vi "Close.vi"(8 "error in (no error)":errorcluster, 11 "VideoMux in":refnum<class "VideoMux.lvclass">) -> (0 "error out":errorcluster)   [LabVIEW 2022 SP3, in "VideoMux.lvlib" / "VideoMux.lvclass"]
uses:
  VideoMux.lvclass
  VideoMux.lvclass/VideoMux.ctl
  <vilib>/IlluminatedG/IG HTTP Server/HTTP Server/Server/Server.lvclass
  <vilib>/ActorFramework/Stop Msg/Stop Msg.lvclass
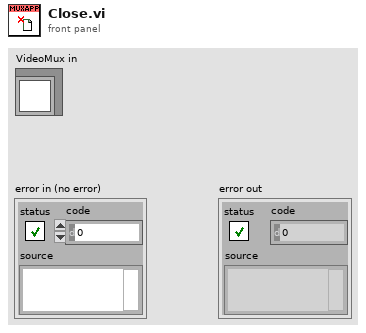
[diagram p1: front panel]
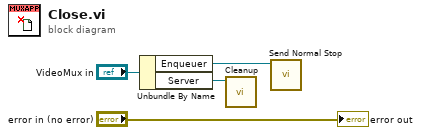
[diagram p0: block diagram]
diagram:
  n1 = Unbundle By Name("VideoMux in") -> ("Enqueuer"=w1:refnum<class "Message Enqueuer.lvclass">, "Server"=w2:refnum<class "Server.lvclass">)
  n2 = call <vilib>:"Cleanup.vi"("Server in"=w2) -> ()  [unwired: 10 in, 1 out]
  n3 = call <vilib>:"Send Normal Stop.vi"("Message Enqueuer"=w1) -> ()  [unwired: 10 in, 1 out]
  "error out" <- "error in (no error)"
